vi "Switch Measurement Channels.vi"(8 "error in (no error)":errorcluster, 9 "Position":u32, 10 "Switch On?":bool, 11 "Measurement in":refnum<class "Measurement.lvclass">) -> (0 "error out":errorcluster)   [LabVIEW 2015, in "Measurement.lvclass"]
uses:
  Measurement.lvclass
  CBTF Applications/Driver Board Testing/Main/Application/Application/Class/typedefs/Instrument Selector -- Enum.ctl
  Classes/Instruments/Relay Control/Switch Executive/Switch Executive.lvclass
  CBTF Applications/Driver Board Testing/Main/Application/Application/Class/Driver Board Test.lvclass
  Test Class/Test Class.lvclass
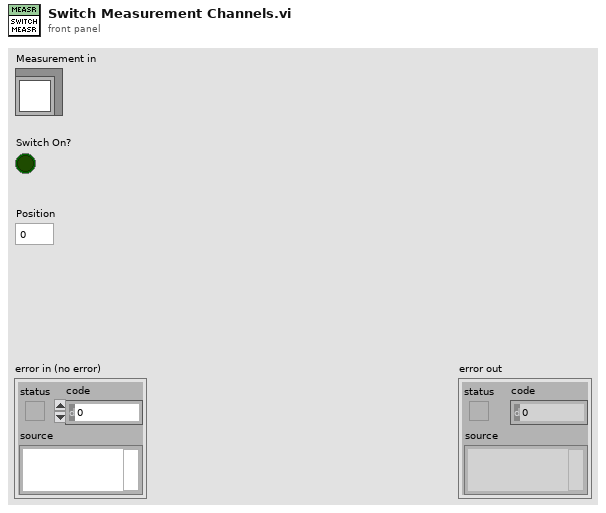
[diagram p1: front panel]
types:
  T1 = typedef "Driver Board Test.lvlib/Driver Board Test.lvclass/Instrument Selector -- Enum.ctl" = enum16{"ACPS1", "ACPS2", "DCPS1", "DCPS2", "DCPS3", "DCLoad1", "DCLoad2", "DPM1", "DPM2", "Switch1", "PXI1Slot2", "PXI1Slot3", "cDAQ1Mod5", "cDAQ1Mod6", "cDAQ1Mod7", "cDAQ1Mod8", "cDAQ1Mod1", "cDAQ1Mod2", "cDAQ1Mod3", "cDAQ1Mod4", "cDAQ2Mod1", "cDAQ2Mod2", "cDAQ2Mod3", "cDAQ2Mod4"}
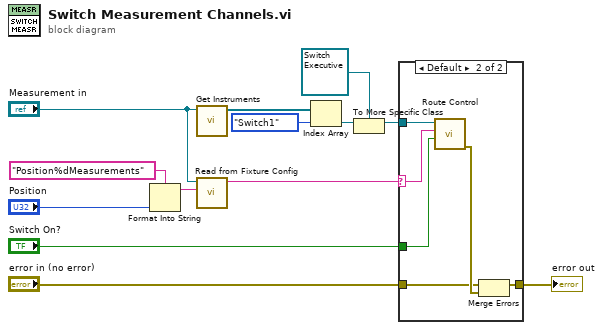
[diagram p0: block diagram]
diagram:
  n1 = Format Into String(format string="Position%dMeasurements", "Position") -> (resulting string=w11:string)  [unwired: 2 in, 1 out]
  n2 = call "Get Instruments.vi"("Test Class in"="Measurement in") -> ("Instruments"=w13:refnum<class "Instrument.lvclass">[])  [unwired: 9 in, 1 out]
  n3 = call-dynamic "Read from Fixture Config.vi"("Key"=w11, "Test Class in"="Measurement in") -> ("Instrument Info"=w12:string)  [unwired: 8 in, 1 out]
  n4 = Index Array(array=w13, index=Instrument_Selector_--_Enum."Switch1" ("Instrument")) -> (element=w8:refnum<class "Instrument.lvclass">)
  n5 = To More Specific Class(target class=refnum<class "Switch Executive.lvclass"> refnum ("Switch Executive.lvlib:Switch Executive.lvclass"), reference=w8) -> (specific class reference=w6:refnum<class "Switch Executive.lvclass">)  [unwired: 1 in, 1 out]
  n6 = case shown="Default" w12 {
    selector: w12 -> [_ w20]
    tunnel: w6 -> [_ w19]
    tunnel: "Switch On?" -> [_ w17]
    tunnel: "error in (no error)" -> [w14 w16]
    tunnel: [w14 w15] -> w1
    frame "" {
    }
    frame Default {
      n7 = call-dynamic "Route Control.vi"("Connect (False)"=w17, "Route Name"=w20, "Switch Executive in"=w19) -> ("error out"=w18:errorcluster)  [unwired: 7 in, 1 out]
      n8 = Merge Errors(w16, w18) -> (w15:errorcluster)
    }
  }
  "error out" <- w1
